vi "Time string to time stamp.vi"(8 "error in (no error)":errorcluster, 10 "Time String":string, 11 "Timestamp Rule Interface in":refnum<class "Timestamp Rule Interface.lvclass">) -> (0 "error out":errorcluster, 2 "Time Stamp":timestamp, 3 "Timestamp Rule Interface out":refnum<class "Timestamp Rule Interface.lvclass">)   [LabVIEW 2020, in "Column Interfaces.lvlib" / "Timestamp Rule Interface.lvclass"]
uses:
  Timestamp Rule Interface.lvclass
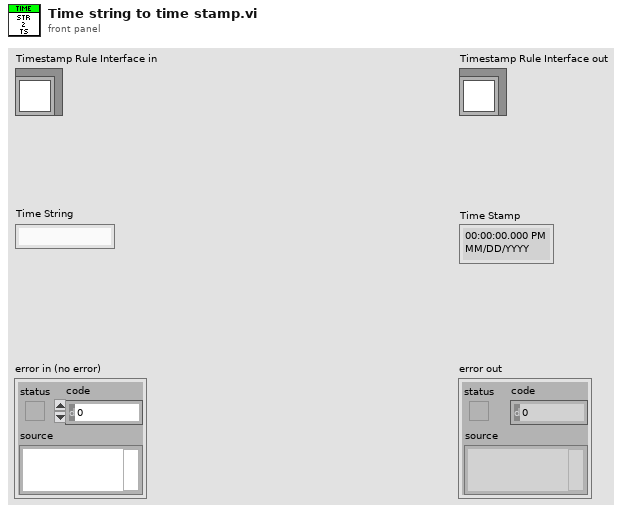
[diagram p1: front panel]
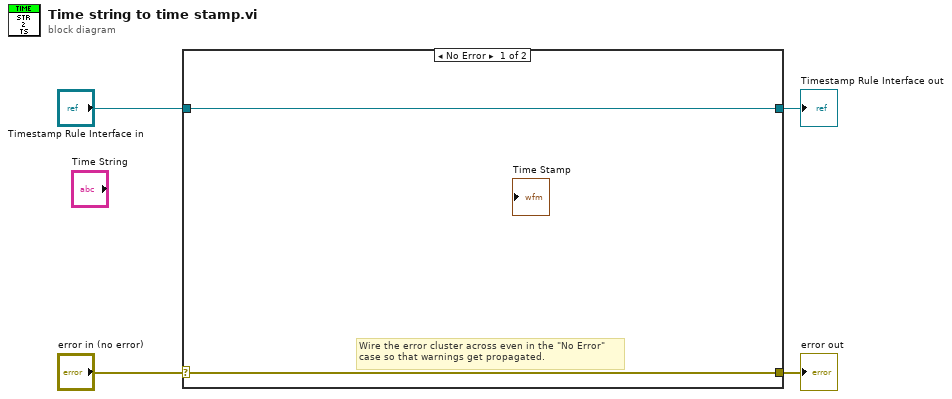
[diagram p0: block diagram]
diagram:
  n1 = case shown="No Error" "error in (no error)" {
    selector: "error in (no error)" -> [w5 w8]
    tunnel: [w5 w8] -> w3
    tunnel: [w6 w7] -> w1
    tunnel: "Timestamp Rule Interface in" -> [w6 w7]
    frame No Error {
      # "Wire the error cluster across even in the \"No Error\"\ncase so that warnings get propagated."
    }
    frame Error {
    }
  }
  "error out" <- w3
  "Timestamp Rule Interface out" <- w1
